vi "PH_Beckhoff_Watchdog.PC _Info.vi"(0 "i ref in":refnum<vi>, 1 "serviceName":string, 2 "Status":T1 items=["no info", "off/false/out", "on/true/in", "Failure", "Alarm", "Status 1", "Status 2", "Status 3"], 3 "Further Information":string="N/A", 4 "no link":bool, 5 "error in":errorcluster) -> (14 "i ref out":refnum<vi>, 19 "error out":errorcluster)   [LabVIEW 2014, in "PH_Beckhoff_Watchdog.lvlib"]
doc: "Within this VI the incoming information is written to own attributes, published at the GUI, and the overall status is calculated, indicated und published."
uses:
  PH_Beckhoff_Watchdog.lvlib
  PH_Basics/PH_StatusHandler/PH_StatusHandler.Status.ctl
  PH_Basics/PH_StatusHandler/PH_StatusHandler.lvlib
  PH_Basics/PH_Common/PH_Common.lvlib
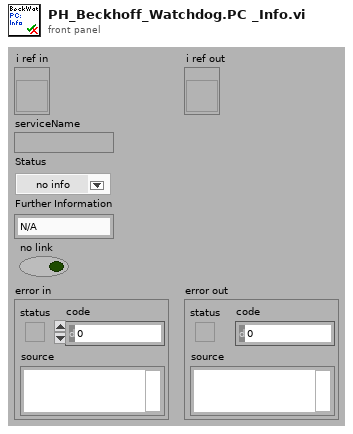
[diagram p1: front panel]
types:
  T1 = typedef "PH_StatusHandler.lvlib/PH_StatusHandler.Status.ctl" = i16
  T2 = typedef "PH_Beckhoff_Watchdog.lvlib/PH_Beckhoff_Watchdog.i attribute.ctl" = cluster{"Info":cluster{"GUI Ref":refnum<vi>, "Status":T1}[]}
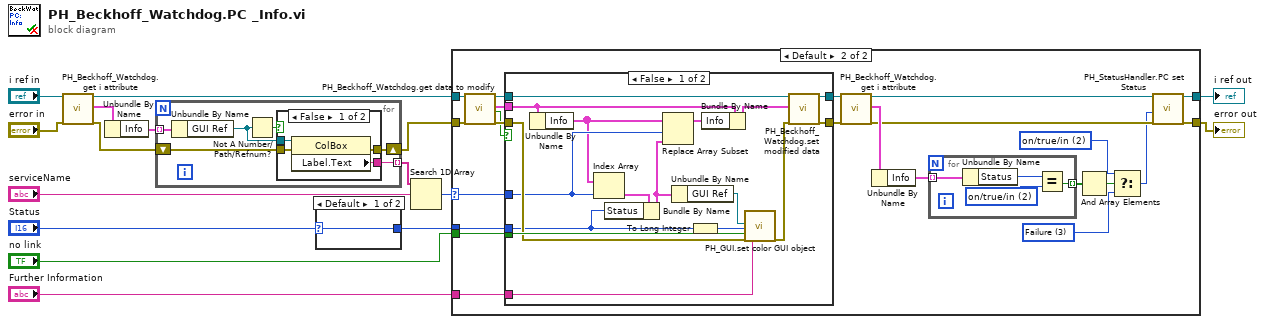
[diagram p0: block diagram]
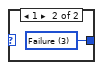
[diagram p2: hidden frame]
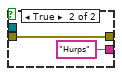
[diagram p5: hidden frame]
diagram:
  n1 = call "PH_Beckhoff_Watchdog.get i attribute.vi"("i ref in"="i ref in", "error in (no error)"="error in") -> ("i ref out"=w4:refnum<vi>, "i attribute"=w6:T2, "error out"=w5:errorcluster)  [unwired: 15 in]
  n2 = Unbundle By Name(w6) -> ("Info"=w10:cluster{"GUI Ref":refnum<vi>, "Status":T1}[])
  n3 = for {
    tunnel: w10 -> [w19] mode=indexing
    shift-right: [w22] -> w7
    shift-left: w5 -> [w21]
    tunnel: [w20] -> w8 mode=indexing
    n4 = Unbundle By Name(w19) -> ("GUI Ref"=w17:refnum<vi>)
    n5 = Not A Number/Path/Refnum?(number/path/refnum=w17) -> (NaN/Path/Refnum?=w18:bool)
    n6 = case shown="False" w18 {
      tunnel: [w26 w28] -> w22
      tunnel: w21 -> [w25 w28]
      tunnel: [w24 "Hurps" ("Label.Text")] -> w20
      tunnel: w17 -> [w23 _]
      frame False {
        n7 = property class="ColBox"(reference=w23, error in=w25) -> (error out=w26:errorcluster, "Label.Text"=w24:string)  [unwired: 1 out]
      }
      frame True {
      }
    }
  }
  n8 = case shown="Default" "Status" {
    selector: "Status" -> [w29 _]
    tunnel: [w29 w30] -> w3
    frame Default {
    }
    frame 1 {
      w30 = T1 3 items=["no info", "off/false/out", "on/true/in", "Failure", "Alarm", "Status 1", "Status 2", "Status 3"] ("Status")
    }
  }
  n9 = Search 1D Array(1D array=w8, element="serviceName") -> (index of element=w9:i32)  [unwired: 1 in]
  n10 = case shown="Default" w9 {
    selector: w9 -> [_ w50]
    tunnel: w4 -> [w32 w55]
    tunnel: [w32 w34] -> w16
    tunnel: [w31 w43] -> w15
    tunnel: w7 -> [w31 w53]
    tunnel: w3 -> [_ w48]
    tunnel: "no link" -> [_ w54]
    tunnel: "Further Information" -> [_ w33]
    frame -1 {
    }
    frame Default {
      w37 = T1 3 items=["no info", "off/false/out", "on/true/in", "Failure", "Alarm", "Status 1", "Status 2", "Status 3"] ("Status")
      w38 = T1 2 items=["no info", "off/false/out", "on/true/in", "Failure", "Alarm", "Status 1", "Status 2", "Status 3"] ("Status")
      n11 = call "PH_Beckhoff_Watchdog.get data to modify.vi"("i ref in"=w55, "error in (no error)"=w53) -> ("i ref out"=w51:refnum<vi>, "i attribute"=w49:T2, "timed out"=w47:bool, "error out"=w52:errorcluster)  [unwired: 14 in]
      n12 = case shown="False" w47 {
        tunnel: w54 -> [w75 _]
        tunnel: [w74 w77] -> w45
        tunnel: w52 -> [w73 w77]
        tunnel: w51 -> [w72 w78]
        tunnel: [w71 w78] -> w46
        tunnel: w50 -> [w70 _]
        tunnel: w49 -> [w68 _]
        tunnel: w48 -> [w64 _]
        tunnel: w33 -> [w63 _]
        frame False {
          n13 = Unbundle By Name(w68) -> ("Info"=w67:cluster{"GUI Ref":refnum<vi>, "Status":T1}[])
          n14 = Index Array(array=w67, index=w70) -> (element=w61:cluster{"GUI Ref":refnum<vi>, "Status":T1})
          n15 = Bundle By Name(cluster=w61, "Status"=w64) -> (w60:cluster{"GUI Ref":refnum<vi>, "Status":T1})
          n16 = Replace Array Subset(array=w67, new element=w60, index=w70) -> (w66:cluster{"GUI Ref":refnum<vi>, "Status":T1}[])
          n17 = Unbundle By Name(w60) -> ("GUI Ref"=w65:refnum<vi>)
          n18 = To Long Integer(number=w64) -> (32bit integer=w62:i32)
          n19 = Bundle By Name(cluster=w68, "Info"=w66) -> (w69:T2)
          n20 = call "PH_GUI.set color GUI object.vi"("GUI object Ref"=w65, "State"=w62, "Blinking? (false)"=w75, "error in (no error)"=w73, "Tip Strip (N/A)"=w63) -> ("error out"=w76:errorcluster)  [unwired: 14 in]
          n21 = call "PH_Beckhoff_Watchdog.set modified data.vi"("i ref in"=w72, "i attribute"=w69, "error in (no error)"=w76) -> ("i ref out"=w71:refnum<vi>, "error out"=w74:errorcluster)  [unwired: 15 in]
        }
        frame True {
        }
      }
      n22 = call "PH_Beckhoff_Watchdog.get i attribute.vi"("i ref in"=w46, "error in (no error)"=w45) -> ("i ref out"=w35:refnum<vi>, "i attribute"=w44:T2, "error out"=w42:errorcluster)  [unwired: 15 in]
      n23 = Unbundle By Name(w44) -> ("Info"=w41:cluster{"GUI Ref":refnum<vi>, "Status":T1}[])
      n24 = for {
        tunnel: w41 -> [w59] mode=indexing
        tunnel: [w56] -> w40 mode=indexing
        w57 = T1 2 items=["no info", "off/false/out", "on/true/in", "Failure", "Alarm", "Status 1", "Status 2", "Status 3"] ("y")
        n25 = Unbundle By Name(w59) -> ("Status"=w58:T1)
        n26 = Equal?(x=w58, y=w57) -> (x = y?=w56:bool)
      }
      n27 = And Array Elements(Boolean array=w40) -> (logical AND=w39:bool)
      n28 = Select(t=w38, s=w39, f=w37) -> (s? t:f=w36:T1)
      n29 = call "PH_StatusHandler.PC set Status.vi"("i ref in"=w35, "Status"=w36, "error in (no error)"=w42) -> ("i ref out"=w34:refnum<vi>, "error out"=w43:errorcluster)  [unwired: 15 in]
    }
  }
  "i ref out" <- w16
  "error out" <- w15
